vi "Station Add.vi"(8 "error in (no error)":errorcluster, 9 "Instruments on Station (none)":T1[](array[typedef]), 10 "Station Record (empty)":T3, 11 "Connection Refnum":T2) -> (0 "error out":errorcluster, 1 "Instruments on Station":T1[](array[typedef]), 2 "New Station Record":T3, 3 "Connection Refnum":T2)   [LabVIEW 2011]
uses:
  Station Record.ctl
  Summitek EXT/ODBC/SQL Controls/Connection Refnum.ctl
  Instruments/Instrument Record.ctl
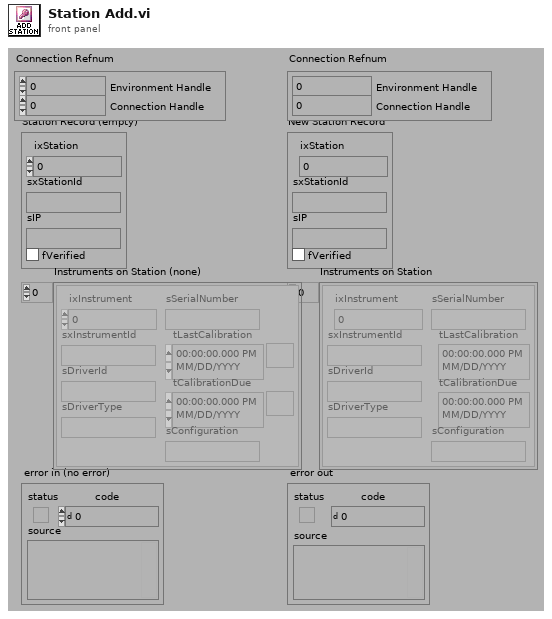
[diagram p1: front panel]
types:
  T1 = typedef "Instrument Record.ctl" = cluster{"ixInstrument":i32, "sxInstrumentId":string, "sDriverId":string, "sDriverType":string, "sSerialNumber":string, "tLastCalibration":timestamp, "tCalibrationDue":timestamp, "sConfiguration":string}
  T2 = typedef "Connection Refnum.ctl" = cluster{"Environment Handle":i32, "Connection Handle":i32}
  T3 = typedef "Station Record.ctl" = cluster{"ixStation":i32, "sxStationId":string, "sIP":string, "fVerified":bool}
  T4 = typedef "Statement Refnum.ctl" = cluster{"Statement Handle":i32, "Parameter Number":u16}
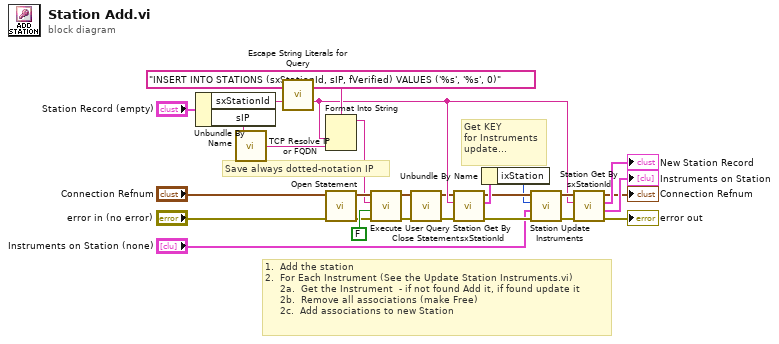
[diagram p0: block diagram]
diagram:
  # "Save always dotted-notation IP"
  # "1.  Add the station\n2.  For Each Instrument (See the Update Station Instruments.vi)\n     2a.  Get the Instrument  - if not found Add it, if found update it\n     2b.  Remove all associations (make Free)\n     2c.  Add associations to new Station"
  # "Get KEY\nfor Instruments\nupdate..."
  n1 = Unbundle By Name("Station Record (empty)") -> ("sxStationId"=w4:string, "sIP"=w8:string)
  n2 = call "TCP Resolve IP or FQDN.vi"("Machine (empty = this machine)"=w8) -> ("Resolved IP or FQDN"=w5:string)
  n3 = call "Escape String Literals for Query.vi"("String"=w4) -> ("escaped String"=w3:string)  [unwired: 1 in, 13 out]
  n4 = Format Into String(format string="INSERT INTO STATIONS (sxStationId, sIP, fVerified) VALUES ('%s', '%s', 0)" ("User Query"), w3, w5) -> (resulting string=w20:string)  [unwired: 2 in, 1 out]
  n5 = call "Open Statement.vi"("error in (no error)"="error in (no error)", "Connection Refnum"="Connection Refnum") -> ("error out"=w23:errorcluster, "Statement Refnum"=w22:T4)  [unwired: 4 out]
  n6 = call "Execute User Query.vi"("error in (no error)"=w23, "Return Data? (f)"=FALSE, "User Query"=w20, "Statement Refnum"=w22) -> ("error out"=w24:errorcluster, "Statement Refnum"=w19:T4)  [unwired: 2 out]
  n7 = call "Close Statement.vi"("error in (no error)"=w24, "Statement Refnum"=w19) -> ("error out"=w18:errorcluster)  [unwired: 5 out]
  n8 = call "Station Get By sxStationId.vi"("error in (no error)"=w18, "sxStationId (\"\")"=w3, "Connection Refnum"="Connection Refnum") -> ("error out"=w12:errorcluster, "Station Record"=w15:T3, "Connection Refnum"=w14:T2)  [unwired: 6 out]
  n9 = Unbundle By Name(w15) -> ("ixStation"=w10:i32)
  n10 = call "Station Update Instruments.vi"("error in (no error)"=w12, "Instruments on Station"="Instruments on Station (none)", "Station KEY (0)"=w10, "Connection Refnum"=w14) -> ("error out"=w11:errorcluster, "Connection Refnum"=w13:T2)  [unwired: 6 out]
  n11 = call "Station Get By sxStationId.vi"("error in (no error)"=w11, "sxStationId (\"\")"=w3, "Connection Refnum"=w13) -> ("error out"=→"error out":errorcluster, "Instruments on Station"=→"Instruments on Station":T1[], "Station Record"=→"New Station Record":T3, "Connection Refnum"=→"Connection Refnum":T2)  [unwired: 5 out]
